vi "AB_RW_Source_Decpwd.vi"(1 "input string":string) -> (0 "output string":string)   [LabVIEW 2020]
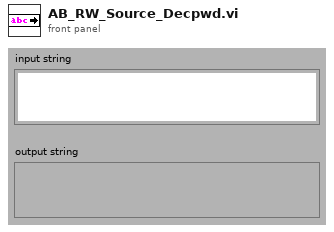
[diagram p1: front panel]
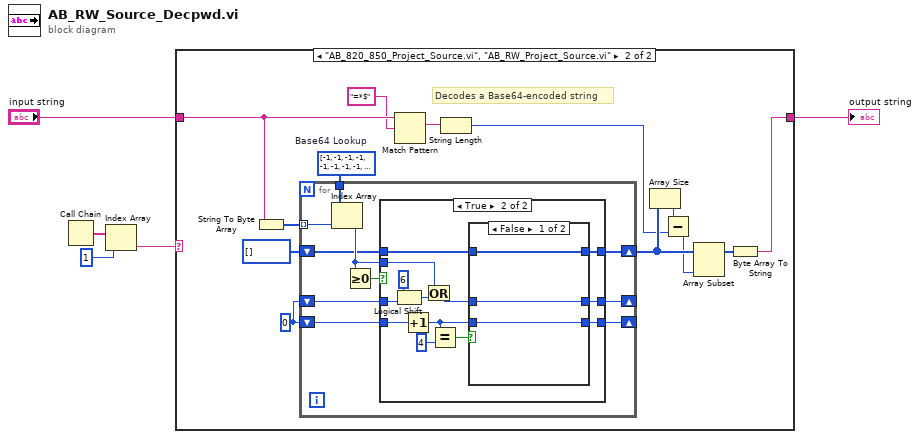
[diagram p0: block diagram]
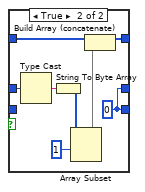
[diagram p4: hidden frame]
diagram:
  n1 = Call Chain() -> (call chain=w2:string[])
  n2 = Index Array(array=w2, index=1) -> (element=w1:string)
  n3 = case shown="\"AB_820_850_Project_Source.vi\", \"AB_RW_Project_Source.vi\"" w1 {
    tunnel: "input string" -> [w6 w15]
    tunnel: [w6 w7] -> w4
    frame "False", Default {
    }
    frame "AB_820_850_Project_Source.vi", "AB_RW_Project_Source.vi" {
      w17 = 0
      w18 = i8[] [-1, -1, -1, -1, -1, -1, -1, -1, -1, -1, -1, -1, -1, -1, -1, -1, -1, -1, -1, -1, -1, -1, -1, -1, -1, -1, -1, -1, -1, -1, -1, -1, -1, -1, -1, -1, -1, -1, -1, -1, -1, -1, -1, 62, -1, -1, -1, 63, 52, 53, 54, 55, 56, 57, 58, 59, 60, 61, -1, -1, -1, 0, -1, -1, -1, 0, 1, 2, 3, 4, 5, 6, 7, 8, 9, 10, 11, 12, 13, 14, 15, 16, 17, 18, 19, 20, 21, 22, 23, 24, 25, -1, -1, -1, -1, -1, -1, 26, 27, 28, 29, 30, 31, 32, 33, 34, 35, 36, 37, 38, 39, 40, 41, 42, 43, 44, 45, 46, 47, 48, 49, 50, 51, -1, -1, -1, -1, -1, -1, -1, -1, -1, -1, -1, -1, -1, -1, -1, -1, -1, -1, -1, -1, -1, -1, -1, -1, -1, -1, -1, -1, -1, -1, -1, -1, -1, -1, -1, -1, -1, -1, -1, -1, -1, -1, -1, -1, -1, -1, -1, -1, -1, -1, -1, -1, -1, -1, -1, -1, -1, -1, -1, -1, -1, -1, -1, -1, -1, -1, -1, -1, -1, -1, -1, -1, -1, -1, -1, -1, -1, -1, -1, -1, -1, -1, -1, -1, -1, -1, -1, -1, -1, -1, -1, -1, -1, -1, -1, -1, -1, -1, -1, -1, -1, -1, -1, -1, -1, -1, -1, -1, -1, -1, -1, -1, -1, -1, -1, -1, -1, -1, -1, -1, -1, -1, -1, -1, -1, -1, -1, -1, -1, -1, -1, -1, -1]  # Base64 Lookup
      # "Decodes a Base64-encoded string"
      n4 = String To Byte Array(string=w15) -> (unsigned byte array=w19:u8[])
      n5 = for {
        tunnel: w19 -> [w29] mode=indexing
        tunnel: w18 -> [w28]
        shift-right: [w22] -> _
        shift-left: w17 -> [w23]
        shift-right: [w27] -> _
        shift-left: w17 -> [w26]
        shift-right: [w20] -> w11
        shift-left: u8[] [] -> [w21]
        n6 = Index Array(array=w28, index=w29) -> (element=w25:i8)
        n7 = Greater Or Equal To 0?(x=w25) -> (x >= 0?=w24:bool)
        n8 = case shown="True" w24 {
          tunnel: w25 -> [_ w45]
          tunnel: w26 -> [w31 w44]
          tunnel: [w31 w38] -> w27
          tunnel: w23 -> [w30 w41]
          tunnel: [w30 w35] -> w22
          tunnel: w21 -> [w32 w34]
          tunnel: [w32 w33] -> w20
          frame False {
          }
          frame True {
            n9 = Logical Shift(y=i16 6, x=w44) -> (x << y=w43:i32)
            n10 = Increment(x=w41) -> (x+1=w36:i32)
            n11 = Or(x=w45, y=w43) -> (x .or. y?=w37:i32)
            n12 = Equal?(x=w36, y=4) -> (x = y?=w39:bool)
            n13 = case shown="False" w39 {
              tunnel: [w48 w56] -> w38
              tunnel: w37 -> [w48 w55]
              tunnel: w36 -> [w47 _]
              tunnel: [w47 w56] -> w35
              tunnel: w34 -> [w46 w51]
              tunnel: [w46 w49] -> w33
              frame False {
              }
              frame True {
                w56 = 0
                n14 = Type Cast(x=w55) -> (*(type *) &x=w54:string)  [unwired: 1 in]
                n15 = String To Byte Array(string=w54) -> (unsigned byte array=w53:u8[])
                n16 = Array Subset(array=w53, index=1) -> (w50:u8[])  [unwired: 1 in]
                n17 = Build Array (concatenate)(w51, w50) -> (w49:u8[])
              }
            }
          }
        }
      }
      n18 = Match Pattern(string=w15, regular expression="=*$") -> (match substring=w13:string)  [unwired: 1 in, 3 out]
      n19 = String Length(string=w13) -> (length=w9:i32)
      n20 = Array Size(array=w11) -> (size(s)=w10:i32)
      n21 = Subtract(x=w10, y=w9) -> (x-y=w8:i32)
      n22 = Array Subset(array=w11, length=w8) -> (w12:u8[])  [unwired: 1 in]
      n23 = Byte Array To String(unsigned byte array=w12) -> (string=w7:string)
    }
  }
  "output string" <- w4
